vi "[SubVI]Matrix_Read.vi"(2 "Model Type":enum16{"DEP", "IND", "SEMI"}(ring)=enum."SEMI") -> (0 "NN Matrix":T2)   [LabVIEW 2018]
uses:
  <vilib>/Analysis/Matrix/Datatypes/RealMatrix.ctl
  <vilib>/Utility/file.llb/Read Delimited Spreadsheet (DBL).vi
  <vilib>/Analysis/Matrix/Numeric/Conversions/Array To Matrix - RA2.vi
  <vilib>/Analysis/Matrix/NI_Matrix.lvlib
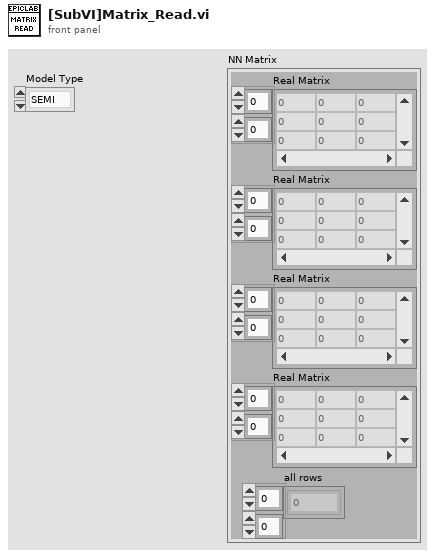
[diagram p1: front panel]
types:
  T1 = typedef "NI_Matrix.lvlib/RealMatrix.ctl" = dbl[][]
  T2 = cluster{"Real Matrix":T1, "Real Matrix":T1, "Real Matrix":T1, "Real Matrix":T1, "all rows":dbl[][]}
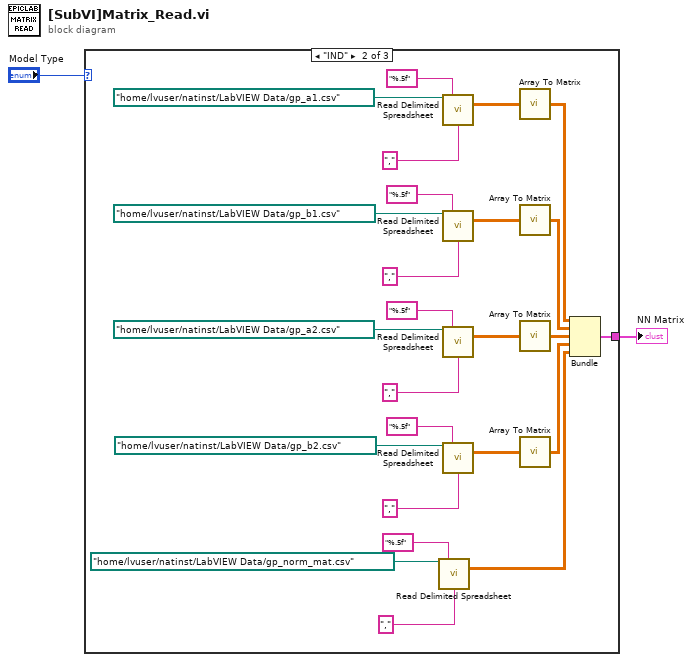
[diagram p0: block diagram]
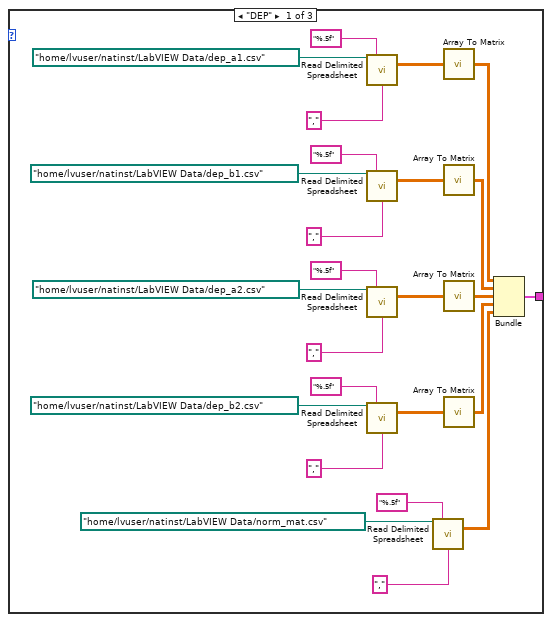
[diagram p2: hidden frame]
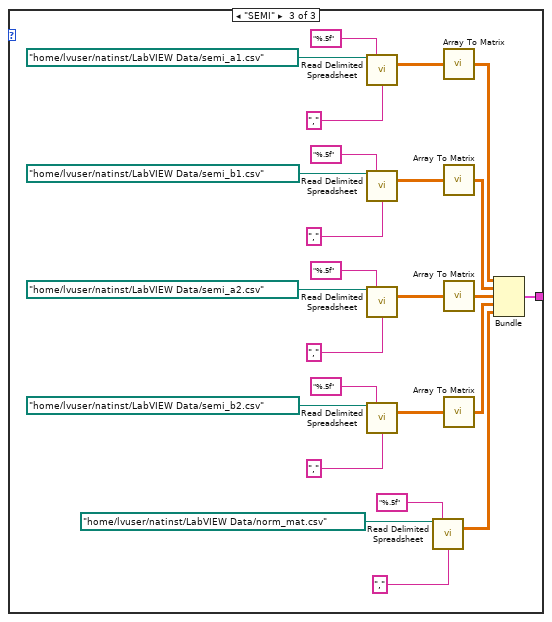
[diagram p3: hidden frame]
diagram:
  n1 = case shown="\"IND\"" "Model Type" {
    tunnel: [w3 w28 w53] -> w1
    frame "DEP" {
      n2 = call-poly <vilib>:"Read Delimited Spreadsheet.vi"("file path (dialog if empty)"=path "/home/lvuser/natinst/LabVIEW Data/dep_a1.csv", "format (%.3f)"="%.5f", "delimiter (\\t)"="," ("delimiter (\\t)")) -> ("all rows"=w19:dbl[][])  [unwired: 7 in, 5 out]
      n3 = call-poly <vilib>:"Read Delimited Spreadsheet.vi"("file path (dialog if empty)"=path "/home/lvuser/natinst/LabVIEW Data/dep_b1.csv", "format (%.3f)"="%.5f", "delimiter (\\t)"="," ("delimiter (\\t)")) -> ("all rows"=w20:dbl[][])  [unwired: 7 in, 5 out]
      n4 = call-poly <vilib>:"Read Delimited Spreadsheet.vi"("file path (dialog if empty)"=path "/home/lvuser/natinst/LabVIEW Data/dep_a2.csv", "format (%.3f)"="%.5f", "delimiter (\\t)"="," ("delimiter (\\t)")) -> ("all rows"=w21:dbl[][])  [unwired: 7 in, 5 out]
      n5 = call-poly <vilib>:"Read Delimited Spreadsheet.vi"("file path (dialog if empty)"=path "/home/lvuser/natinst/LabVIEW Data/dep_b2.csv", "format (%.3f)"="%.5f", "delimiter (\\t)"="," ("delimiter (\\t)")) -> ("all rows"=w22:dbl[][])  [unwired: 7 in, 5 out]
      n6 = call-poly <vilib>:"Read Delimited Spreadsheet.vi"("file path (dialog if empty)"=path "/home/lvuser/natinst/LabVIEW Data/norm_mat.csv", "format (%.3f)"="%.5f", "delimiter (\\t)"="," ("delimiter (\\t)")) -> ("all rows"=w27:dbl[][])  [unwired: 7 in, 5 out]
      n7 = call-poly <vilib>:"Array To Matrix.vi"("Real 2D Array"=w19) -> ("Real Matrix"=w23:T1)
      n8 = call-poly <vilib>:"Array To Matrix.vi"("Real 2D Array"=w20) -> ("Real Matrix"=w24:T1)
      n9 = call-poly <vilib>:"Array To Matrix.vi"("Real 2D Array"=w21) -> ("Real Matrix"=w25:T1)
      n10 = call-poly <vilib>:"Array To Matrix.vi"("Real 2D Array"=w22) -> ("Real Matrix"=w26:T1)
      n11 = Bundle("Real Matrix"=w23, "Real Matrix"=w24, "Real Matrix"=w25, "Real Matrix"=w26, "all rows"=w27) -> (w3:T2)  [unwired: 1 in]
    }
    frame "IND" {
      n12 = call-poly <vilib>:"Read Delimited Spreadsheet.vi"("file path (dialog if empty)"=path "/home/lvuser/natinst/LabVIEW Data/gp_norm_mat.csv", "format (%.3f)"="%.5f", "delimiter (\\t)"="," ("delimiter (\\t)")) -> ("all rows"=w29:dbl[][])  [unwired: 7 in, 5 out]
      n13 = call-poly <vilib>:"Read Delimited Spreadsheet.vi"("file path (dialog if empty)"=path "/home/lvuser/natinst/LabVIEW Data/gp_a1.csv", "format (%.3f)"="%.5f", "delimiter (\\t)"="," ("delimiter (\\t)")) -> ("all rows"=w46:dbl[][])  [unwired: 7 in, 5 out]
      n14 = call-poly <vilib>:"Read Delimited Spreadsheet.vi"("file path (dialog if empty)"=path "/home/lvuser/natinst/LabVIEW Data/gp_b1.csv", "format (%.3f)"="%.5f", "delimiter (\\t)"="," ("delimiter (\\t)")) -> ("all rows"=w45:dbl[][])  [unwired: 7 in, 5 out]
      n15 = call-poly <vilib>:"Read Delimited Spreadsheet.vi"("file path (dialog if empty)"=path "/home/lvuser/natinst/LabVIEW Data/gp_a2.csv", "format (%.3f)"="%.5f", "delimiter (\\t)"="," ("delimiter (\\t)")) -> ("all rows"=w41:dbl[][])  [unwired: 7 in, 5 out]
      n16 = call-poly <vilib>:"Read Delimited Spreadsheet.vi"("file path (dialog if empty)"=path "/home/lvuser/natinst/LabVIEW Data/gp_b2.csv", "format (%.3f)"="%.5f", "delimiter (\\t)"="," ("delimiter (\\t)")) -> ("all rows"=w37:dbl[][])  [unwired: 7 in, 5 out]
      n17 = call-poly <vilib>:"Array To Matrix.vi"("Real 2D Array"=w46) -> ("Real Matrix"=w36:T1)
      n18 = call-poly <vilib>:"Array To Matrix.vi"("Real 2D Array"=w45) -> ("Real Matrix"=w35:T1)
      n19 = call-poly <vilib>:"Array To Matrix.vi"("Real 2D Array"=w41) -> ("Real Matrix"=w34:T1)
      n20 = call-poly <vilib>:"Array To Matrix.vi"("Real 2D Array"=w37) -> ("Real Matrix"=w33:T1)
      n21 = Bundle("Real Matrix"=w36, "Real Matrix"=w35, "Real Matrix"=w34, "Real Matrix"=w33, "all rows"=w29) -> (w28:T2)  [unwired: 1 in]
    }
    frame "SEMI" {
      n22 = call-poly <vilib>:"Read Delimited Spreadsheet.vi"("file path (dialog if empty)"=path "/home/lvuser/natinst/LabVIEW Data/semi_a1.csv", "format (%.3f)"="%.5f", "delimiter (\\t)"="," ("delimiter (\\t)")) -> ("all rows"=w71:dbl[][])  [unwired: 7 in, 5 out]
      n23 = call-poly <vilib>:"Read Delimited Spreadsheet.vi"("file path (dialog if empty)"=path "/home/lvuser/natinst/LabVIEW Data/semi_b1.csv", "format (%.3f)"="%.5f", "delimiter (\\t)"="," ("delimiter (\\t)")) -> ("all rows"=w70:dbl[][])  [unwired: 7 in, 5 out]
      n24 = call-poly <vilib>:"Read Delimited Spreadsheet.vi"("file path (dialog if empty)"=path "/home/lvuser/natinst/LabVIEW Data/semi_a2.csv", "format (%.3f)"="%.5f", "delimiter (\\t)"="," ("delimiter (\\t)")) -> ("all rows"=w66:dbl[][])  [unwired: 7 in, 5 out]
      n25 = call-poly <vilib>:"Read Delimited Spreadsheet.vi"("file path (dialog if empty)"=path "/home/lvuser/natinst/LabVIEW Data/semi_b2.csv", "format (%.3f)"="%.5f", "delimiter (\\t)"="," ("delimiter (\\t)")) -> ("all rows"=w62:dbl[][])  [unwired: 7 in, 5 out]
      n26 = call-poly <vilib>:"Read Delimited Spreadsheet.vi"("file path (dialog if empty)"=path "/home/lvuser/natinst/LabVIEW Data/norm_mat.csv", "format (%.3f)"="%.5f", "delimiter (\\t)"="," ("delimiter (\\t)")) -> ("all rows"=w54:dbl[][])  [unwired: 7 in, 5 out]
      n27 = call-poly <vilib>:"Array To Matrix.vi"("Real 2D Array"=w71) -> ("Real Matrix"=w61:T1)
      n28 = call-poly <vilib>:"Array To Matrix.vi"("Real 2D Array"=w70) -> ("Real Matrix"=w60:T1)
      n29 = call-poly <vilib>:"Array To Matrix.vi"("Real 2D Array"=w66) -> ("Real Matrix"=w59:T1)
      n30 = call-poly <vilib>:"Array To Matrix.vi"("Real 2D Array"=w62) -> ("Real Matrix"=w58:T1)
      n31 = Bundle("Real Matrix"=w61, "Real Matrix"=w60, "Real Matrix"=w59, "Real Matrix"=w58, "all rows"=w54) -> (w53:T2)  [unwired: 1 in]
    }
  }
  "NN Matrix" <- w1
